vi "Multimeter.vi"(1 "GPIB address":string="22") -> (0 "DC Voltage":dbl=-3.22473e-08 format="%.2e")   [LabVIEW 2013]
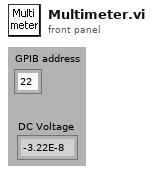
[diagram p1: front panel]
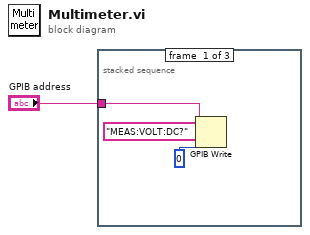
[diagram p0: block diagram]
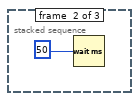
[diagram p2: hidden frame]
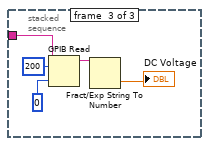
[diagram p3: hidden frame]
diagram:
  n1 = stacked-sequence {
    tunnel: "GPIB address" -> [w4 _ w10]
    frame #0 {
      n2 = GPIB Write(0:w4, 1:"MEAS:VOLT:DC?", 2:0) -> ()  [unwired: 2 in, 2 out]
    }
    frame #1 {
      n3 = Wait (ms)(milliseconds to wait=50) -> ()  [unwired: 1 out]
    }
    frame #2 {
      n4 = GPIB Read(0:w10, 1:200, 2:0) -> (5:w9:string)  [unwired: 2 in, 2 out]
      n5 = Fract/Exp String To Number(string=w9) -> (number=→"DC Voltage":dbl)  [unwired: 3 in, 1 out]
    }
  }
